vi "autonomous sonar (basic).vi"   [LabVIEW 2010, in "Tank Robot.lvrbt"]
uses:
  Tank Robot.lvrbt
  <vilib>/NXT/Block Support/NXT_InputPort.ctl
  <vilib>/NXT/NXTIO Xnodes/AddressXNode/NXTIOAddress.xnode
  <vilib>/NXT/Subs/MotorXNode.DC Motor Type.ctl
  <vilib>/NXT/Subs/MotorXNode.2DCMotor.ctl
  <vilib>/NXT/Subs/LVHSConnector.ctl
  <vilib>/NXT/NXTIO Xnodes/NXTIOXNode/NXTIO.xnode
  <vilib>/NXT/Dual Mode Library/Sensors/Sonar_cm.vi
  <vilib>/NXT/Dual Mode Library/prims/inRangeAndCoerce/inRangeAndCoerce_int.vi
  <vilib>/NXT/Dual Mode Library/Display/drawNumber.vi
  <vilib>/NXT/Dual Mode Library/prims/inRangeAndCoerce/inRangeAndCoerce_float.vi
  <vilib>/NXT/NXTIO Xnodes/NXTIONodeSubVIs/TETRIX IO Move DC Motors.vi
types:
  T1 = typedef "NXT_InputPort.ctl" = u8
  T2 = typedef "MotorXNode.DC Motor Type.ctl" = enum16{"DC Motor"}
  T3 = cluster{"DC Motor":T2, "Address":i16, "Address":i16}
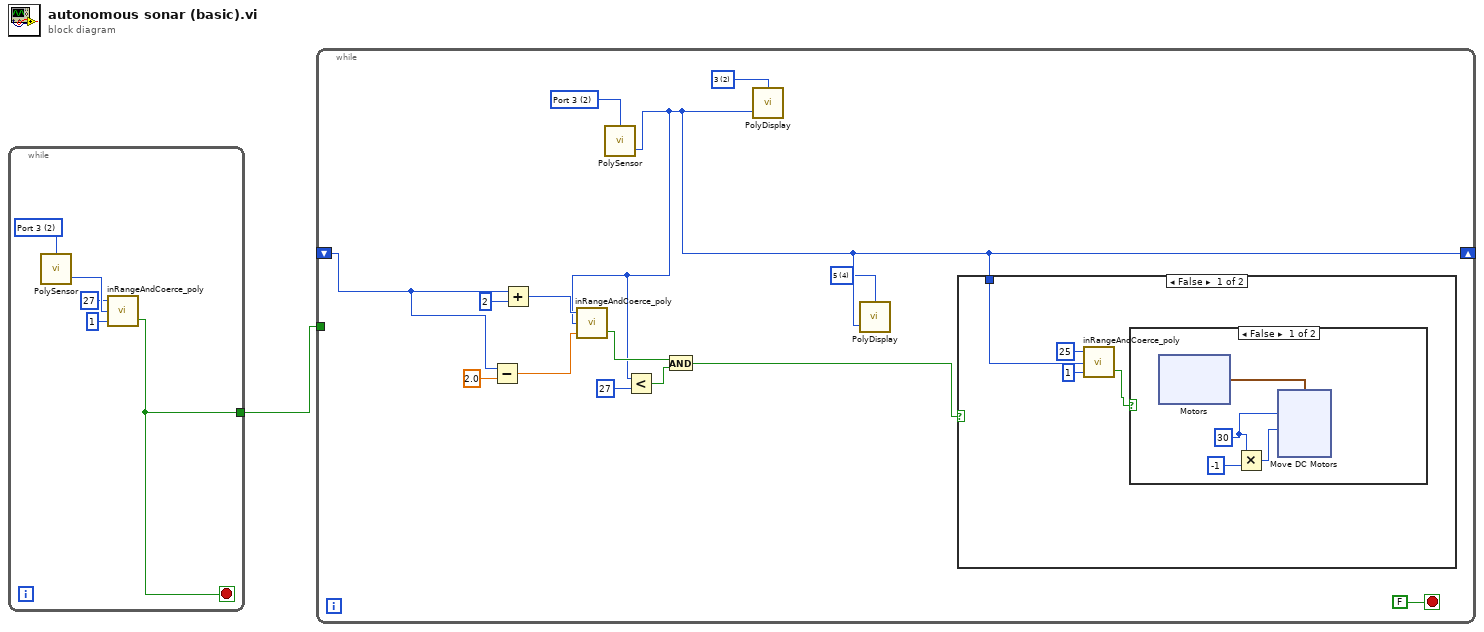
[diagram p0: block diagram]
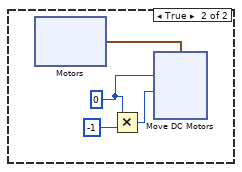
[diagram p2: hidden frame]
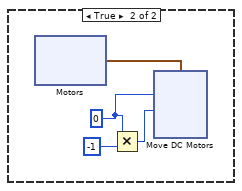
[diagram p3: hidden frame]
diagram:
  n1 = while {
    tunnel: [w2] -> w1
    stop <- w2 stop-if-true
    w6 = T1 2 items=["Port 1", "Port 2", "Port 3", "Port 4"] ("Port (Port 4)")
    n2 = call-poly <vilib>:"PolySensor.vi"("Port (Port 4)"=w6) -> ("Distance (cm)"=w5:i16)  [unwired: 2 in, 1 out]
    n3 = call-poly <vilib>:"inRangeAndCoerce_poly.vi"("lower limit"=1, "x"=w5, "upper limit"=27) -> ("In Range?"=w2:bool)  [unwired: 1 out]
  }
  n4 = while {
    shift-right: [w8] -> _
    shift-left: _ -> [w14]
    tunnel: w1 -> [_]
    stop <- FALSE stop-if-true
    w7 = i16 4 items=["1", "2", "3", "4", "5", "6", "7", "8"] ("Line")
    w18 = i16 2 items=["1", "2", "3", "4", "5", "6", "7", "8"] ("Line")
    w19 = T1 2 items=["Port 1", "Port 2", "Port 3", "Port 4"] ("Port (Port 4)")
    n5 = Subtract(x=w14, y=2.0) -> (x-y=w13:dbl)
    n6 = Add(x=w14, y=i16 2) -> (x+y=w16:i16)
    n7 = call-poly <vilib>:"PolySensor.vi"("Port (Port 4)"=w19) -> ("Distance (cm)"=w8:i16)  [unwired: 2 in, 1 out]
    n8 = call-poly <vilib>:"inRangeAndCoerce_poly.vi"("lower limit"=w13, "x"=w8, "upper limit"=w16) -> ("In Range?"=w10:bool)  [unwired: 1 out]
    n9 = Less?(x=w8, y=i16 27) -> (x < y?=w12:bool)
    n10 = And(x=w10, y=w12) -> (x .and. y?=w9:bool)
    n11 = call-poly <vilib>:"PolyDisplay.vi"("number"=w8, "Line"=w18) -> ()  [unwired: 2 in, 1 out]
    n12 = call-poly <vilib>:"PolyDisplay.vi"("number"=w8, "Line"=w7) -> ()  [unwired: 2 in, 1 out]
    n13 = case shown="False" w9 {
      tunnel: w8 -> [w24 _]
      frame False {
        n14 = call-poly <vilib>:"inRangeAndCoerce_poly.vi"("lower limit"=1, "x"=w24, "upper limit"=25) -> ("In Range?"=w21:bool)  [unwired: 1 out]
        n15 = case shown="False" w21 {
          frame False {
            w27 = 30
            n16 = xnode "Motors"() -> ("DC Motor"=w28:T3)
            n17 = Multiply(x=w27, y=-1) -> (x*y=w25:i32)
            n18 = xnode "Move DC Motors"("Power/Speed 2"=w25, "Power/Speed 1"=w27, "Motors"=w28) -> ()  [unwired: 1 in, 1 out]
          }
          frame True {
            w42 = 0
            n19 = xnode "Motors"() -> ("DC Motor"=w43:T3)
            n20 = Multiply(x=w42, y=-1) -> (x*y=w40:i32)
            n21 = xnode "Move DC Motors"("Power/Speed 2"=w40, "Power/Speed 1"=w42, "Motors"=w43) -> ()  [unwired: 1 in, 1 out]
          }
        }
      }
      frame True {
        w57 = 0
        n22 = xnode "Motors"() -> ("DC Motor"=w58:T3)
        n23 = Multiply(x=w57, y=-1) -> (x*y=w55:i32)
        n24 = xnode "Move DC Motors"("Power/Speed 2"=w55, "Power/Speed 1"=w57, "Motors"=w58) -> ()  [unwired: 1 in, 1 out]
      }
    }
  }
